vi "Actor Core.vi"(8 "error in":errorcluster, 11 "Sensor View in":refnum<class "Sensor View.lvclass">) -> (0 "error out":errorcluster, 3 "Actor out":refnum<class "Actor.lvclass">)   [LabVIEW 2013, in "Sensor View.lvlib" / "Sensor View.lvclass"]
doc: "(<B>Filename</B>: Actor Framework.lvlib:Actor.lvclass:Actor Core.vi)\n\nReceives messages to the actor, reacts to them, and initiates any error handling that may shut the actor down.\n\nDescendant classes may override this VI to append parallel tasks for the actor to complete while it handles messages. Overrides use the Call Parent Method node."
uses:
  Sensor View.lvclass
  <vilib>/ActorFramework/Actor/Actor.lvclass
  Resources/UI Controls/Tiles.ctl
  Resources/UI Controls/Tile.ctl
  Resources/UI Controls/Add Tile.ctl
  Resources/UI Controls/Delete Frame.ctl
  Sensor View.lvclass/Sensor View.ctl
  <vilib>/ActorFramework/Actor/Actor.lvclass/Actor.ctl
  <vilib>/ActorFrameworkMVC/View Actor/View Actor.lvclass
  <vilib>/ActorFramework/Message Enqueuer/Message Enqueuer.lvclass/Message Enqueuer.ctl
  Sensor View Messages/Set Frame Visibility Msg/Set Frame Visibility Msg.lvclass/Set Frame Visibility Msg.ctl
  Sensor View Messages/Update Tiles Msg/Update Tiles Msg.lvclass/Update Tiles Msg.ctl
  <vilib>/ActorFrameworkMVC/UI Controller Messages/Move Splitter Msg/Move Splitter Msg.lvclass/Move Splitter Msg.ctl
  <vilib>/Utility/miscctls.llb/LVPositionTypeDef.ctl
  <vilib>/ActorFrameworkMVC/UI Controller Messages/Move Subpanel Msg/Move Subpanel Msg.lvclass/Move Subpanel Msg.ctl
  <vilib>/ActorFrameworkMVC/UI Controller Messages/Insert Subpanel Msg/Insert Subpanel Msg.lvclass/Insert Subpanel Msg.ctl
  Models/Edit Sensor Model Messages/Set Framed Sensor Path Msg/Set Framed Sensor Path Msg.lvclass/Set Framed Sensor Path Msg.ctl
  Sensor View Messages/Move Frame Msg/Move Frame Msg.lvclass/Move Frame Msg.ctl
  Models/Sensor Model Messages/Set Framed Project Path Msg/Set Framed Project Path Msg.lvclass/Set Framed Project Path Msg.ctl
  <vilib>/ActorFramework/Message Enqueuer/Init from Existing Queue.vi
  <vilib>/ActorFramework/Message Enqueuer/Enqueue.vi
  <vilib>/ActorFramework/Message Priority Queue/Priority Enqueue.vi
  <vilib>/ActorFramework/Message Enqueuer/Message Enqueuer.lvclass
  Sensor View Messages/Set Frame Visibility Msg/Set Frame Visibility Msg.lvclass
  Sensor View Messages/Update Tiles Msg/Update Tiles Msg.lvclass
  Sensor View Messages/Move In Previous Page Msg/Move In Previous Page Msg.lvclass
  Sensor View Messages/Move In Next Page Msg/Move In Next Page Msg.lvclass
  <vilib>/ActorFrameworkMVC/UI Controller Messages/Move Splitter Msg/Move Splitter Msg.lvclass
  <vilib>/ActorFrameworkMVC/UI Controller Messages/Move Subpanel Msg/Move Subpanel Msg.lvclass
  <vilib>/ActorFrameworkMVC/UI Controller Messages/Insert Subpanel Msg/Insert Subpanel Msg.lvclass
  Models/Main Model Messages/List Project File Msg/List Project File Msg.lvclass
  Models/Main Model Messages/Update Project Number Msg/Update Project Number Msg.lvclass
  Models/Create Sensor Model Messages/Reinitialize All Msg/Reinitialize All Msg.lvclass
  Models/Create Sensor Model Messages/Key Focus Msg/Key Focus Msg.lvclass
  Sensor View Messages/Move Out Next Page Msg/Move Out Next Page Msg.lvclass
  Models/Sensor Model Messages/Next Page Msg/Next Page Msg.lvclass
  Sensor View Messages/Move Out Previous Page Msg/Move Out Previous Page Msg.lvclass
  Models/Sensor Model Messages/Previous Page Msg/Previous Page Msg.lvclass
  Models/Edit Sensor Model Messages/Set Framed Sensor Path Msg/Set Framed Sensor Path Msg.lvclass
  Models/Edit Sensor Model Messages/Initialized Edit Sensor Msg/Initialized Edit Sensor Msg.lvclass
  Sensor View Messages/Move Frame Msg/Move Frame Msg.lvclass
  Models/Sensor Model Messages/Set Framed Project Path Msg/Set Framed Project Path Msg.lvclass
  <vilib>/ActorFrameworkMVC/View Actor Messages/Get Model Enqueuer Msg/Get Model Enqueuer Msg.lvclass
  <vilib>/ActorFrameworkMVC/UI Controller Messages/Get Model Actor Enqueuer Msg/Get Model Actor Enqueuer Msg.lvclass
panel:
  in  "Frame":T1
  in  "Previous Button":bool
  in  "Next Button":bool
  in  "Add Tile":T2
  out "Tiles":T3
  in  "Back":bool
  # "传感器"
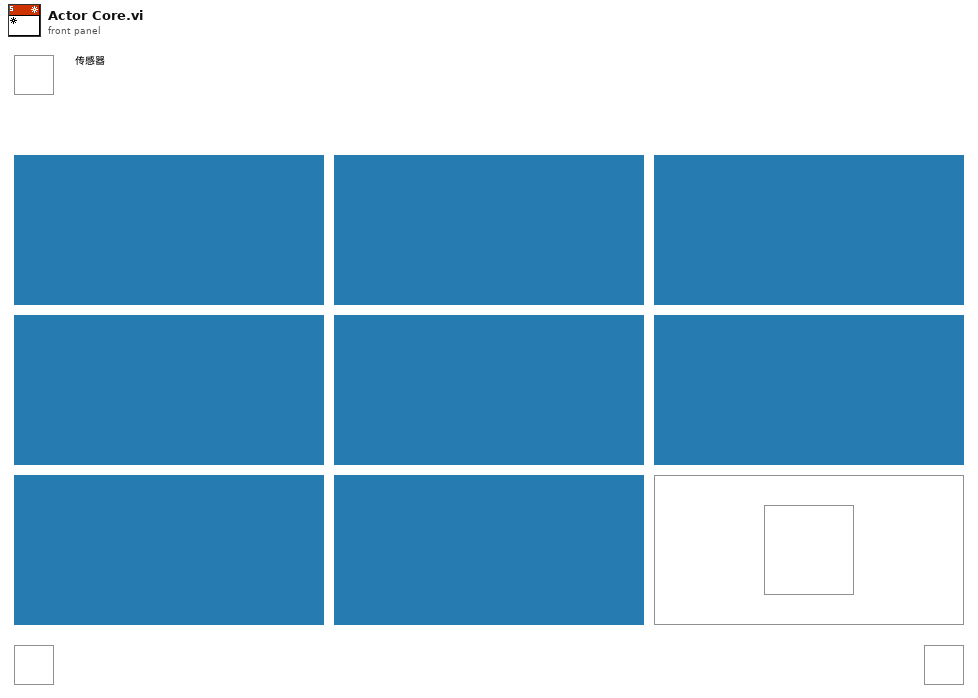
[diagram p1: front panel]
types:
  T1 = typedef "Delete Frame.ctl" = bool
  T2 = typedef "Add Tile.ctl" = bool
  T3 = typedef "Tiles.ctl" = cluster{"Tile 1":T4, "Tile 2":T4, "Tile 3":T4, "Tile 4":T4, "Tile 5":T4, "Tile 6":T4, "Tile 7":T4, "Tile 8":T4}
  T4 = typedef "Tile.ctl" = cluster{"Name":string, "Spec":string, "File Path":string}
  T5 = typedef "Sensor View.lvlib/Sensor View.lvclass/Events.ctl" = cluster{"Update Tiles Info":refnum<user-event>, "Set Previous Button Visibility":refnum<user-event>, "Set Next Button Visibility":refnum<user-event>, "Move In Previous":refnum<user-event>, "Move In Next":refnum<user-event>}
  T6 = typedef "LVPositionTypeDef.ctl" = cluster{"Left":i32, "Top":i32}
  T7 = enum8{"Enabled", "Disabled", "Disabled and Grayed Out"}
  T8 = typedef "Info Cluster.ctl" = cluster{"Name":string, "Spec":string, "File Path":string}
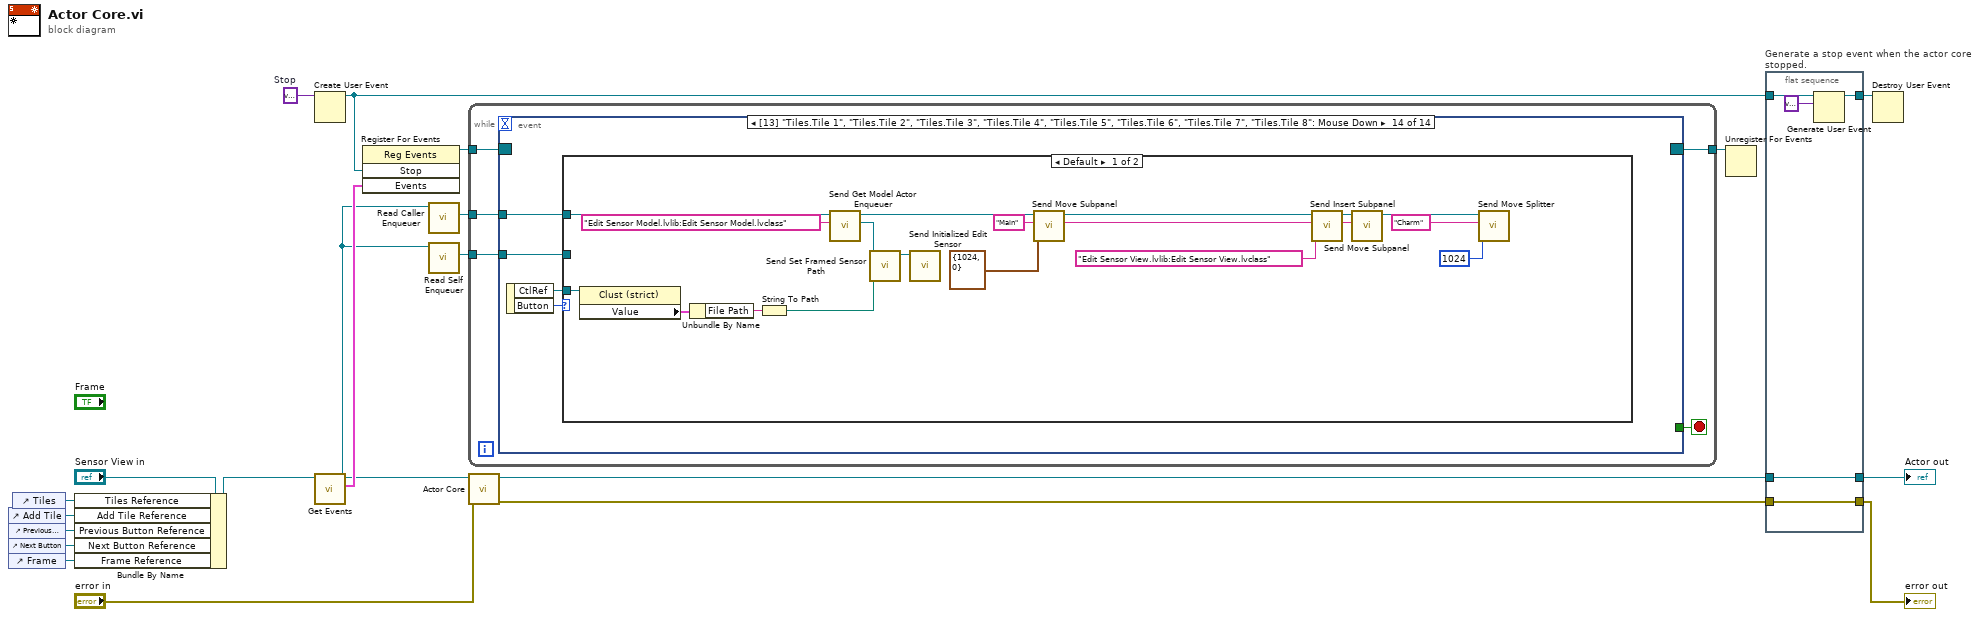
[diagram p0: block diagram]
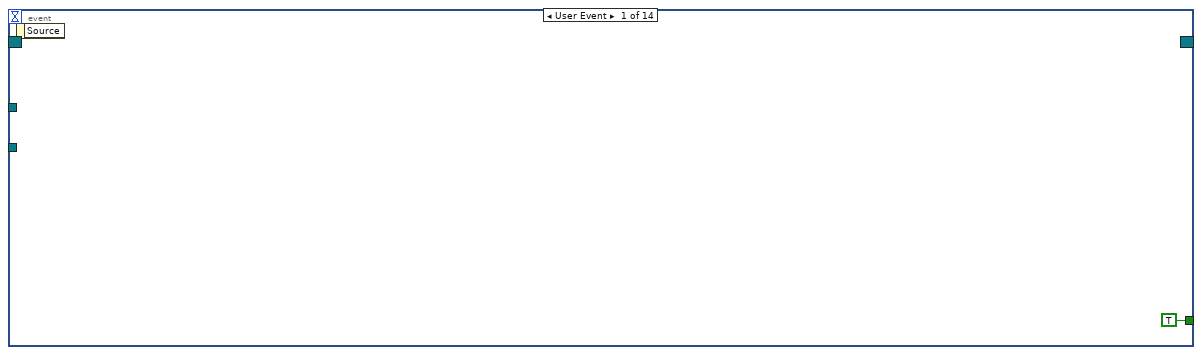
[diagram p2: hidden frame]
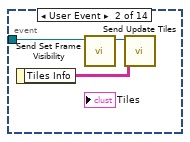
[diagram p3: hidden frame]
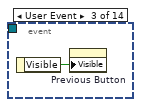
[diagram p4: hidden frame]
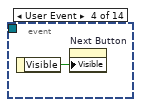
[diagram p5: hidden frame]
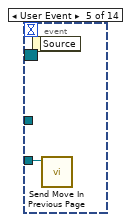
[diagram p6: hidden frame]
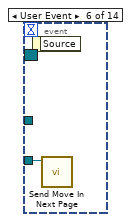
[diagram p7: hidden frame]
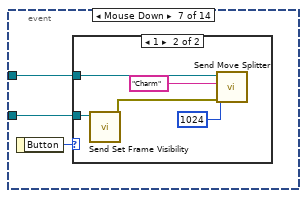
[diagram p8: hidden frame]
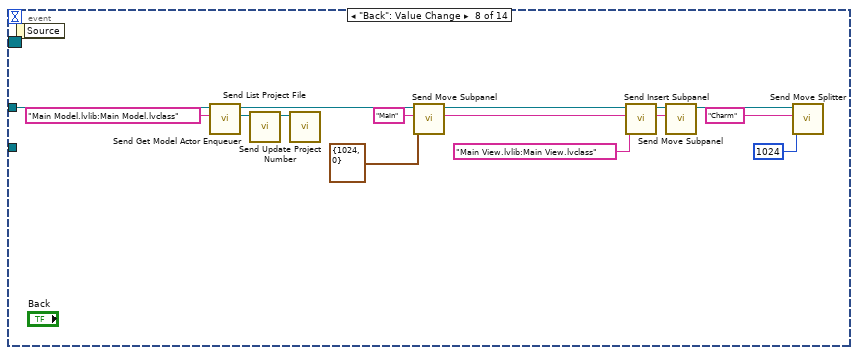
[diagram p10: hidden frame]
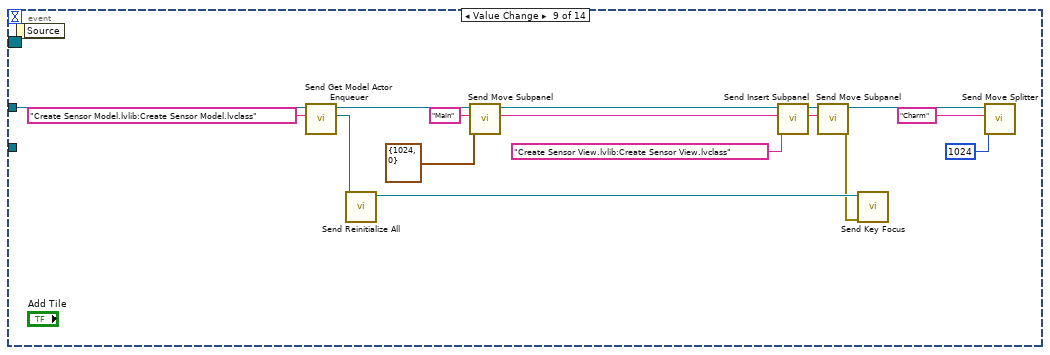
[diagram p11: hidden frame]
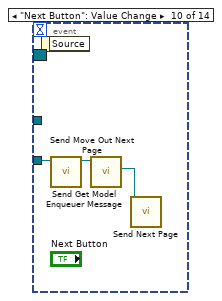
[diagram p12: hidden frame]
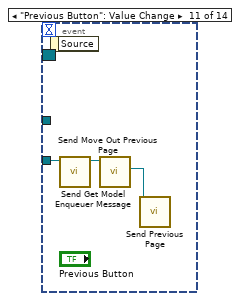
[diagram p13: hidden frame]
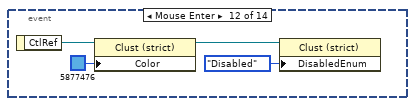
[diagram p14: hidden frame]
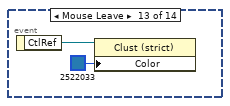
[diagram p15: hidden frame]
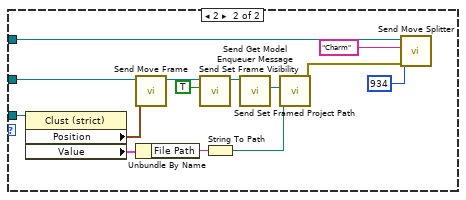
[diagram p16: hidden frame]
diagram:
  w21 = variant  # Stop
  n1 = control-ref of="Add Tile"() -> (w4:refnum<vi>)
  n2 = control-ref of="Previous Button"() -> (w5:refnum<vi>)
  n3 = control-ref of="Next Button"() -> (w6:refnum<vi>)
  n4 = control-ref of="Frame"() -> (w7:refnum<vi>)
  n5 = control-ref of="Tiles"() -> (w8:refnum<vi>)
  n6 = Bundle By Name(cluster="Sensor View in", "Tiles Reference"=w8, "Add Tile Reference"=w4, "Previous Button Reference"=w5, "Next Button Reference"=w6, "Frame Reference"=w7) -> (w9:refnum<class "Sensor View.lvclass">)
  n7 = Create User Event(user event datatype=w21) -> (user event=w12:refnum<user-event>)  [unwired: 1 in, 1 out]
  n8 = call "Get Events.vi"("Sensor View in"=w9) -> ("Events"=w11:T5, "Sensor View out"=w3:refnum<class "Sensor View.lvclass">)  [unwired: 9 in]
  n9 = register-events(w12, w11) -> (reference out=w13:refnum<event-registration>)  [unwired: 2 in, 1 out]
  n10 = call <vilib>:"Read Caller Enqueuer.vi"("Actor"=w3) -> ("Caller Enqueuer"=w2:refnum<class "Message Enqueuer.lvclass">)  [unwired: 10 in]
  n11 = call <vilib>:"Read Self Enqueuer.vi"("Actor"=w3) -> ("Self Enqueuer"=w1:refnum<class "Message Enqueuer.lvclass">)  [unwired: 10 in]
  n12 = while {
    tunnel: [w26] -> w10
    tunnel: w13 -> [w24]
    tunnel: w2 -> [w23]
    tunnel: w1 -> [w22]
    stop <- w25 stop-if-true
    n13 = event shown="[13] \"Tiles.Tile 1\", \"Tiles.Tile 2\", \"Tiles.Tile 3\", \"Tiles.Tile 4\", \"Tiles.Tile 5\", \"Tiles.Tile 6\", \"Tiles.Tile 7\", \"Tiles.Tile 8\": Mouse Down" {
      selector: w24 -> [_ _ _ _ _ _ _ _ _ _ _ _ _ _]
      dyn-events: [_ _ _ _ _ _ _ _ _ _ _ _ _ _] -> w26
      timeout: _ -> [_ _ _ _ _ _ _ _ _ _ _ _ _ _]
      tunnel: [TRUE _ _ _ _ _ _ _ _ _ _ _ _ _] -> w25
      tunnel: w23 -> [_ _ _ _ _ _ w37 w44 w60 _ _ _ _ w82]
      tunnel: w22 -> [_ w30 _ _ w33 w34 w35 _ _ w71 w74 _ _ w83]
      event User Event {
        n14 = event-data() -> ()  [unwired: 1 in, 1 out]
      }
      event User Event {
        n15 = event-data() -> ("Tiles Info"=w28:string[][])  [unwired: 1 in]
        n16 = call "Send Set Frame Visibility.vi"("Message Enqueuer"=w30) -> ("Message Enqueuer out"=w29:refnum<class "Message Enqueuer.lvclass">)  [unwired: 9 in, 1 out]
        n17 = call "Send Update Tiles.vi"("Sensor Tiles Info"=w28, "Message Enqueuer"=w29) -> ()  [unwired: 8 in, 2 out]
      }
      event User Event {
        n18 = event-data() -> ("Visible"=w31:bool)  [unwired: 1 in]
        n19 = property on="Previous Button" class="Bool"("Visible"=w31) -> ()  [unwired: 2 in, 2 out]
      }
      event User Event {
        n20 = event-data() -> ("Visible"=w32:bool)  [unwired: 1 in]
        n21 = property on="Next Button" class="Bool"("Visible"=w32) -> ()  [unwired: 2 in, 2 out]
      }
      event User Event {
        n22 = event-data() -> ()  [unwired: 1 in, 1 out]
        n23 = call "Send Move In Previous Page.vi"("Message Enqueuer"=w33) -> ()  [unwired: 9 in, 2 out]
      }
      event User Event {
        n24 = event-data() -> ()  [unwired: 1 in, 1 out]
        n25 = call "Send Move In Next Page.vi"("Message Enqueuer"=w34) -> ()  [unwired: 9 in, 2 out]
      }
      event Mouse Down {
        n26 = event-data() -> ("Button"=w36:u16)  [unwired: 1 in]
        n27 = case shown="1" w36 {
          tunnel: w37 -> [_ w42]
          tunnel: w35 -> [_ w39]
          frame 0, Default {
          }
          frame 1 {
            n28 = call "Send Set Frame Visibility.vi"("Message Enqueuer"=w39) -> ("error out"=w38:errorcluster)  [unwired: 9 in, 1 out]
            n29 = call <vilib>:"Send Move Splitter.vi"("error in (no error)"=w38, "Splitter Position"=1024, "Splitter Name"="Charm", "Message Enqueuer"=w42) -> ()  [unwired: 6 in, 2 out]
          }
        }
      }
      event "Back": Value Change {
        w52 = "Main" ("Subpanel Name")
        n30 = event-data() -> ()  [unwired: 1 in, 1 out]
        n31 = call <vilib>:"Send Get Model Actor Enqueuer.vi"("Model Name"="Main Model.lvlib:Main Model.lvclass", "Message Enqueuer in"=w44) -> ("Reply"=w47:refnum<class "Message Enqueuer.lvclass">, "Message Enqueuer out"=w43:refnum<class "Message Enqueuer.lvclass">)  [unwired: 6 in, 2 out]
        n32 = call "Send List Project File.vi"("Message Enqueuer"=w47) -> ("Message Enqueuer out"=w46:refnum<class "Message Enqueuer.lvclass">)  [unwired: 9 in, 1 out]
        n33 = call "Send Update Project Number.vi"("Message Enqueuer"=w46) -> ()  [unwired: 9 in, 2 out]
        n34 = call <vilib>:"Send Move Subpanel.vi"("Position (0,0)"=T6 {"Left"=1024, "Top"=0}, "Subpanel Name"=w52, "Message Enqueuer"=w43) -> ("Message Enqueuer out"=w55:refnum<class "Message Enqueuer.lvclass">)  [unwired: 7 in, 1 out]
        n35 = call <vilib>:"Send Insert Subpanel.vi"("View Name"="Main View.lvlib:Main View.lvclass", "Subpanel Name"=w52, "Message Enqueuer"=w55) -> ("Message Enqueuer out"=w53:refnum<class "Message Enqueuer.lvclass">)  [unwired: 7 in, 1 out]
        n36 = call <vilib>:"Send Move Subpanel.vi"("Subpanel Name"=w52, "Message Enqueuer"=w53) -> ("Message Enqueuer out"=w51:refnum<class "Message Enqueuer.lvclass">)  [unwired: 8 in, 1 out]
        n37 = call <vilib>:"Send Move Splitter.vi"("Splitter Position"=1024, "Splitter Name"="Charm", "Message Enqueuer"=w51) -> ()  [unwired: 7 in, 2 out]
      }
      event Value Change {
        w66 = "Main" ("Subpanel Name")
        n38 = event-data() -> ()  [unwired: 1 in, 1 out]
        n39 = call <vilib>:"Send Get Model Actor Enqueuer.vi"("Model Name"="Create Sensor Model.lvlib:Create Sensor Model.lvclass", "Message Enqueuer in"=w60) -> ("Reply"=w58:refnum<class "Message Enqueuer.lvclass">, "Message Enqueuer out"=w59:refnum<class "Message Enqueuer.lvclass">)  [unwired: 6 in, 2 out]
        n40 = call "Send Reinitialize All.vi"("Message Enqueuer"=w58) -> ("Message Enqueuer out"=w57:refnum<class "Message Enqueuer.lvclass">)  [unwired: 9 in, 1 out]
        n41 = call <vilib>:"Send Move Subpanel.vi"("Position (0,0)"=T6 {"Left"=1024, "Top"=0}, "Subpanel Name"=w66, "Message Enqueuer"=w59) -> ("Message Enqueuer out"=w69:refnum<class "Message Enqueuer.lvclass">)  [unwired: 7 in, 1 out]
        n42 = call <vilib>:"Send Insert Subpanel.vi"("View Name"="Create Sensor View.lvlib:Create Sensor View.lvclass", "Subpanel Name"=w66, "Message Enqueuer"=w69) -> ("Message Enqueuer out"=w67:refnum<class "Message Enqueuer.lvclass">)  [unwired: 7 in, 1 out]
        n43 = call <vilib>:"Send Move Subpanel.vi"("Subpanel Name"=w66, "Message Enqueuer"=w67) -> ("error out"=w56:errorcluster, "Message Enqueuer out"=w65:refnum<class "Message Enqueuer.lvclass">)  [unwired: 8 in]
        n44 = call "Send Key Focus.vi"("error in (no error)"=w56, "Message Enqueuer"=w57) -> ()  [unwired: 8 in, 2 out]
        n45 = call <vilib>:"Send Move Splitter.vi"("Splitter Position"=1024, "Splitter Name"="Charm", "Message Enqueuer"=w65) -> ()  [unwired: 7 in, 2 out]
      }
      event "Next Button": Value Change {
        n46 = event-data() -> ()  [unwired: 1 in, 1 out]
        n47 = call "Send Move Out Next Page.vi"("Message Enqueuer"=w71) -> ("Message Enqueuer out"=w70:refnum<class "Message Enqueuer.lvclass">)  [unwired: 9 in, 1 out]
        n48 = call <vilib>:"Send Get Model Enqueuer Message.vi"("Message Enqueuer in"=w70) -> ("Reply"=w72:refnum<class "Message Enqueuer.lvclass">)  [unwired: 7 in, 3 out]
        n49 = call "Send Next Page.vi"("Message Enqueuer"=w72) -> ()  [unwired: 9 in, 2 out]
      }
      event "Previous Button": Value Change {
        n50 = event-data() -> ()  [unwired: 1 in, 1 out]
        n51 = call "Send Move Out Previous Page.vi"("Message Enqueuer"=w74) -> ("Message Enqueuer out"=w73:refnum<class "Message Enqueuer.lvclass">)  [unwired: 9 in, 1 out]
        n52 = call <vilib>:"Send Get Model Enqueuer Message.vi"("Message Enqueuer in"=w73) -> ("Reply"=w75:refnum<class "Message Enqueuer.lvclass">)  [unwired: 7 in, 3 out]
        n53 = call "Send Previous Page.vi"("Message Enqueuer"=w75) -> ()  [unwired: 9 in, 2 out]
      }
      event Mouse Enter {
        n54 = event-data() -> ("CtlRef"=w76:refnum<vi>)  [unwired: 1 in]
        n55 = property class="Clust (strict)"(reference=w76, "Color"=u32 5877476) -> (reference out=w78:refnum<vi>)  [unwired: 1 in, 1 out]
        n56 = property class="Clust (strict)"(reference=w78, "DisabledEnum"=T7."Disabled" ("Disabled")) -> ()  [unwired: 1 in, 2 out]
      }
      event Mouse Leave {
        n57 = event-data() -> ("CtlRef"=w80:refnum<vi>)  [unwired: 1 in]
        n58 = property class="Clust (strict)"(reference=w80, "Color"=u32 2522033) -> ()  [unwired: 1 in, 2 out]
      }
      event Mouse Down {
        n59 = event-data() -> ("CtlRef"=w85:refnum<vi>, "Button"=w84:u16)  [unwired: 1 in]
        n60 = case shown="Default" w84 {
          tunnel: w85 -> [w99 w116]
          tunnel: w83 -> [_ w115]
          tunnel: w82 -> [w102 w111]
          frame Default {
            w90 = "Main" ("Subpanel Name")
            n61 = property class="Clust (strict)"(reference=w99) -> ("Value"=w98:T4)  [unwired: 1 in, 2 out]
            n62 = Unbundle By Name(w98) -> ("File Path"=w97:string)
            n63 = String To Path(string=w97) -> (path=w96:path)
            n64 = call <vilib>:"Send Get Model Actor Enqueuer.vi"("Model Name"="Edit Sensor Model.lvlib:Edit Sensor Model.lvclass", "Message Enqueuer in"=w102) -> ("Reply"=w100:refnum<class "Message Enqueuer.lvclass">, "Message Enqueuer out"=w86:refnum<class "Message Enqueuer.lvclass">)  [unwired: 6 in, 2 out]
            n65 = call "Send Set Framed Sensor Path.vi"("Framed Sensor Path"=w96, "Message Enqueuer"=w100) -> ("Message Enqueuer out"=w95:refnum<class "Message Enqueuer.lvclass">)  [unwired: 8 in, 1 out]
            n66 = call "Send Initialized Edit Sensor.vi"("Message Enqueuer"=w95) -> ()  [unwired: 9 in, 2 out]
            n67 = call <vilib>:"Send Move Subpanel.vi"("Position (0,0)"=T6 {"Left"=1024, "Top"=0}, "Subpanel Name"=w90, "Message Enqueuer"=w86) -> ("Message Enqueuer out"=w87:refnum<class "Message Enqueuer.lvclass">)  [unwired: 7 in, 1 out]
            n68 = call <vilib>:"Send Insert Subpanel.vi"("View Name"="Edit Sensor View.lvlib:Edit Sensor View.lvclass", "Subpanel Name"=w90, "Message Enqueuer"=w87) -> ("Message Enqueuer out"=w89:refnum<class "Message Enqueuer.lvclass">)  [unwired: 7 in, 1 out]
            n69 = call <vilib>:"Send Move Subpanel.vi"("Subpanel Name"=w90, "Message Enqueuer"=w89) -> ("Message Enqueuer out"=w91:refnum<class "Message Enqueuer.lvclass">)  [unwired: 8 in, 1 out]
            n70 = call <vilib>:"Send Move Splitter.vi"("Splitter Position"=1024, "Splitter Name"="Charm", "Message Enqueuer"=w91) -> ()  [unwired: 7 in, 2 out]
          }
          frame 2 {
            n71 = property class="Clust (strict)"(reference=w116) -> ("Position"=w114:T6, "Value"=w107:T8)  [unwired: 1 in, 2 out]
            n72 = call "Send Move Frame.vi"("Position"=w114, "Message Enqueuer"=w115) -> ("Message Enqueuer out"=w113:refnum<class "Message Enqueuer.lvclass">)  [unwired: 8 in, 1 out]
            n73 = Unbundle By Name(w107) -> ("File Path"=w106:string)
            n74 = call "Send Set Frame Visibility.vi"("Visible (F)"=TRUE, "Message Enqueuer"=w113) -> ("Message Enqueuer out"=w108:refnum<class "Message Enqueuer.lvclass">)  [unwired: 8 in, 1 out]
            n75 = String To Path(string=w106) -> (path=w105:path)
            n76 = call <vilib>:"Send Get Model Enqueuer Message.vi"("Message Enqueuer in"=w108) -> ("Reply"=w103:refnum<class "Message Enqueuer.lvclass">)  [unwired: 7 in, 3 out]
            n77 = call "Send Set Framed Project Path.vi"("Framed Project Path"=w105, "Message Enqueuer"=w103) -> ("error out"=w104:errorcluster)  [unwired: 8 in, 1 out]
            n78 = call <vilib>:"Send Move Splitter.vi"("error in (no error)"=w104, "Splitter Position"=934, "Splitter Name"="Charm", "Message Enqueuer"=w111) -> ()  [unwired: 6 in, 2 out]
          }
        }
      }
    }
  }
  n79 = call-parent "Actor Core.vi"("error in"="error in", "View Actor in"=w3) -> ("error out"=w16:errorcluster, "Actor out"=w17:refnum<class "Actor.lvclass">)  [unwired: 8 in]
  n80 = Unregister For Events(event registration refnum=w10) -> ()  [unwired: 1 in, 1 out]
  n81 = flat-sequence "Generate a stop event when the actor core stopped." {
    tunnel: w12 -> [w121]
    tunnel: [w119] -> w20
    tunnel: w17 -> [w118]
    tunnel: w16 -> [w117]
    tunnel: [w118] -> w15
    tunnel: [w117] -> w14
    frame #0 {
      n82 = Generate User Event(user event=w121, event data cluster=variant ("event data")) -> (user event out=w119:refnum<user-event>)  [unwired: 2 in, 1 out]
    }
  }
  n83 = Destroy User Event(user event=w20) -> ()  [unwired: 1 in, 1 out]
  "error out" <- w14
  "Actor out" <- w15
